vi "CPP_SolAE_Plot_Many_Channels.vi"() -> (5 "Plug in titles":string[](array[string]), 7 "Plug in values":string[](array[string]))   [LabVIEW 2021]
uses:
  <vilib>/Analysis/2dsp.llb/Decimate (single shot, DBL).vi
  07834b75-344c-4d4c-a66e-07bf327eec95.vi
  Globals/Meas_global.vi
  <vilib>/Analysis/NI_AALBase.lvlib
  <vilib>/Analysis/NI_AALPro.lvlib
panel:
  in  "decimating factor":i32=400
  in  "Tab Control":T1(tab)
  out "XY Graph":cluster{"Time (s)":dbl[], "Voltage":dbl[]}[](graph)
  out "XY Graph 2":cluster{"Time (s)":dbl[], "Voltage":dbl[]}[](graph)
  out "XY Graph 3":cluster{"Time (s)":dbl[], "Voltage":dbl[]}[](graph)
  out "XY Graph 4":cluster{"Time (s)":dbl[], "Voltage":dbl[]}[](graph)
  out "XY Graph 5":cluster{"Time (s)":dbl[], "Voltage":dbl[]}[](graph)
  out "XY Graph 6":cluster{"Time (s)":dbl[], "Voltage":dbl[]}[](graph)
  in  "Display:":enum16{"Show All", "My Choice", "Hide All"}(ring)
  in  "Plot:":enum16{"Eng. Units", "Voltages"}(ring)
  # "Channel"
  # "Value"
  # "Voltage"
  # "StdDev(V)"
  # "Name"
  # "Symbol"
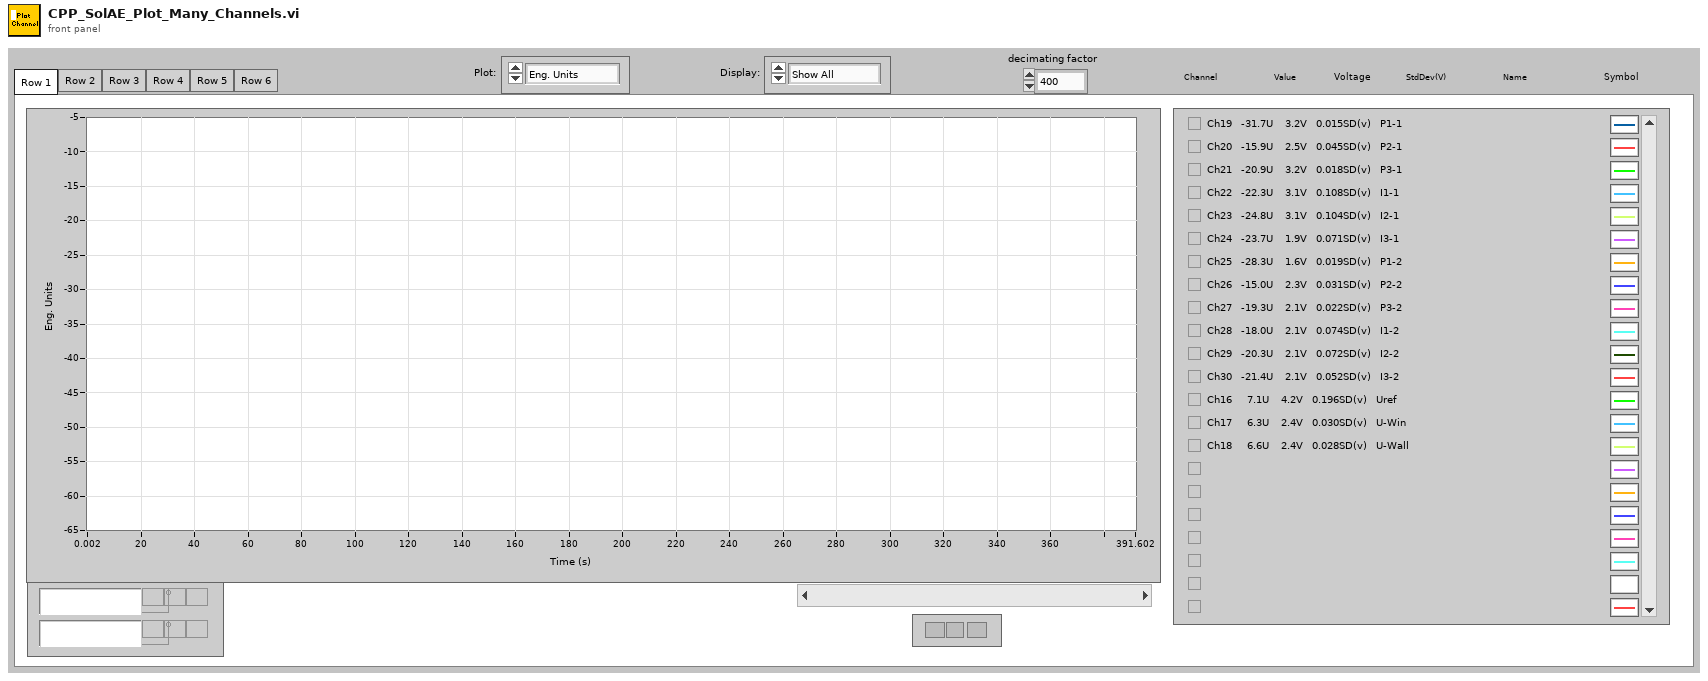
[diagram p1: front panel]
types:
  T1 = enum32{"Row 1", "Row 2", "Row 3", "Row 4", "Row 5", "Row 6"}
  T2 = typedef "Analysis_info_cluster.ctl" = cluster{"Colour":u32, "Inst type":T3, "Inst name":string, "Symbol":string, "Code name":string, "Extra Info":string, "Inst Array":T4, "Extra Titles":string[], "Extra Values":string[], "U":dbl, "u^2":dbl, "u^3":dbl, "u^4":dbl, "Skew_u":dbl, "Kurt_u":dbl, "Sd Error in Mean":dbl, "% u'/U":dbl, "X":dbl, "Y":dbl, "Z":dbl, "Timescale integral Estimate":dbl, "Sd Error in Variance":dbl, "Calib File":path, "Calib Constants":dbl[], "Output Position":bool, "Stats":enum16{"None", "Basic", "Full"}, "Av Sampling Rate":dbl, "Av No of Samples":dbl, "Total Meas Time (s)":dbl, "ADAM Ch Name":string, "Max value":dbl, "Min value":dbl, "Req Sample Rate Hz":dbl, "Sync Delay Time (s)":dbl, "Ch No":i16, "Device":string, "Use Latest Calib":bool, "Port":string, "Metadata Ch Names":string[], "Metadata Ch Values":string[], "Label":string}
  T3 = typedef "Inst_type.ctl" = enum16{"Raw voltage", "Raw with zero offsetting", "Propeller anemometer", "Pressure Transducer", "Pitot-static tube", "Hot wire", "Cross wire 1", "Cross wire 2", "Generic Linear", "Generic Polynomial", "Generic BackPoly", "Fast FID", "Thermocouple", "Cold wire", "Pulsed Wire", "LDA Vel", "LDA Tran time", "LDA Arr time", "Microphone"}
  T4 = typedef "Instrument_Array.ctl" = enum16{"PWA", "LDA", "Analogue"}
  T5 = typedef "Time_Trace_Cluster.ctl" = cluster{"Weighting":dbl[], "Voltage":dbl[], "Eng Values":dbl[]}
  T6 = cluster{"Decimated Array":dbl[], "Decimated Array":dbl[]}
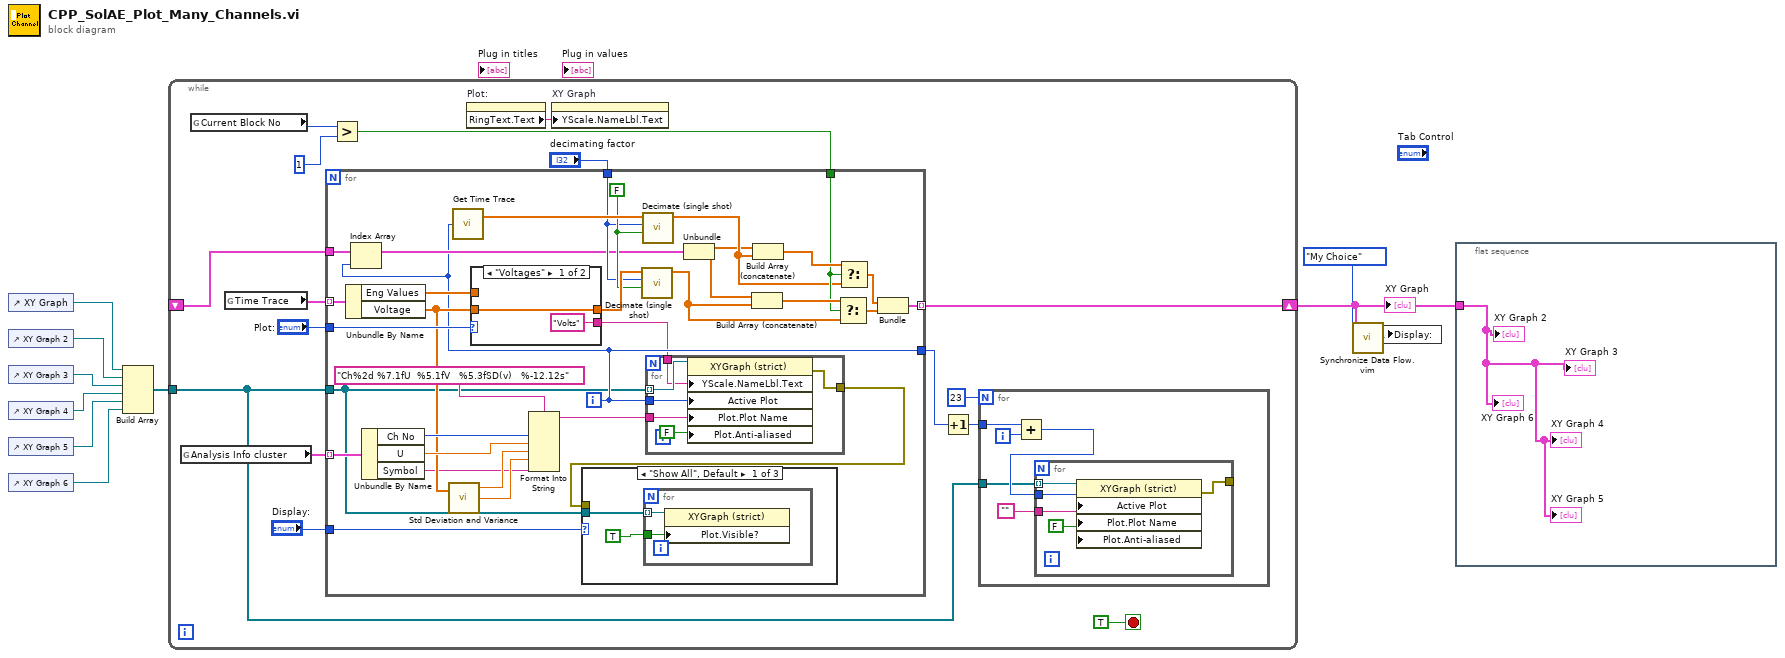
[diagram p0: block diagram]
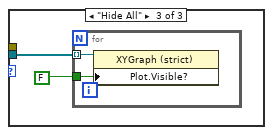
[diagram p3: hidden frame]
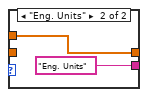
[diagram p4: hidden frame]
diagram:
  n1 = control-ref of="XY Graph"() -> (w7:refnum<vi>)
  n2 = control-ref of="XY Graph 2"() -> (w6:refnum<vi>)
  n3 = control-ref of="XY Graph 3"() -> (w5:refnum<vi>)
  n4 = control-ref of="XY Graph 4"() -> (w4:refnum<vi>)
  n5 = control-ref of="XY Graph 5"() -> (w3:refnum<vi>)
  n6 = control-ref of="XY Graph 6"() -> (w2:refnum<vi>)
  n7 = Build Array(w7, w6, w5, w4, w3, w2) -> (w1:refnum<vi>[])
  n8 = while {
    shift-right: [w21] -> w8
    shift-left: _ -> [w13]
    tunnel: w1 -> [w11]
    stop <- TRUE stop-if-true
    n9 = global read "Meas_global.vi" "Analysis Info cluster"() -> (w26:T2[])
    n10 = global read "Meas_global.vi" "Current Block No"() -> (w16:i32)
    n11 = global read "Meas_global.vi" "Time Trace"() -> (w23:T5[])
    n12 = Greater?(x=w16, y=1) -> (0:w12:bool)
    n13 = for {
      tunnel: [w51] -> w21 mode=indexing
      tunnel: w26 -> [w69] mode=indexing
      tunnel: "Plot:" -> [w68]
      tunnel: "Display:" -> [w57]
      tunnel: w23 -> [w56] mode=indexing
      tunnel: [w39] -> w19
      tunnel: "decimating factor" -> [w52]
      tunnel: w13 -> [w50]
      tunnel: w12 -> [w45]
      tunnel: w11 -> [w38]
      i -> [w39]
      w53 = FALSE ("averaging")
      n14 = Unbundle By Name(w56) -> ("Eng Values"=w63:dbl[], "Voltage"=w62:dbl[])
      n15 = Index Array(array=w50, index=w39) -> (element=w40:T6)
      n16 = Unbundle By Name(w69) -> ("Ch No"=w67:i16, "U"=w66:dbl, "Symbol"=w59:string)
      n17 = call <vilib>:"Std Deviation and Variance.vi"("X"=w62) -> ("mean"=w61:dbl, "standard deviation"=w60:dbl)  [unwired: 1 in, 1 out]
      n18 = call "Get Time Trace.vi"("Channel Index"=w39) -> ("Time (s)"=w55:dbl[])  [unwired: 1 out]
      n19 = case shown="\"Voltages\"" w68 {
        tunnel: [w85 w87] -> w54
        tunnel: w62 -> [w85 _]
        tunnel: w63 -> [_ w87]
        tunnel: ["Volts" "Eng. Units"] -> w37
        frame "Voltages" {
        }
        frame "Eng. Units" {
        }
      }
      n20 = Format Into String(format string="Ch%2d %7.1fU  %5.1fV   %5.3fSD(v)   %-12.12s", w67, w66, w61, w60, w59) -> (resulting string=w65:string)  [unwired: 2 in, 1 out]
      n21 = call-poly <vilib>:"Decimate (single shot).vi"("averaging"=w53, "decimating factor"=w52, "X"=w54) -> ("Decimated Array"=w47:dbl[])  [unwired: 7 in, 1 out]
      n22 = call-poly <vilib>:"Decimate (single shot).vi"("averaging"=w53, "decimating factor"=w52, "X"=w55) -> ("Decimated Array"=w42:dbl[])  [unwired: 7 in, 1 out]
      n23 = for {
        tunnel: w65 -> [w75]
        tunnel: [w74] -> w58
        tunnel: w39 -> [w71]
        tunnel: w38 -> [w73] mode=indexing
        tunnel: w37 -> [w70]
        n24 = property class="XYGraph (strict)"(reference=w73, "YScale.NameLbl.Text"=w70, "Active Plot"=w71, "Plot.Plot Name"=w75, "Plot.Anti-aliased"=FALSE) -> (error out=w74:errorcluster)  [unwired: 1 in, 1 out]
      }
      n25 = case shown="\"Show All\", Default" w57 {
        tunnel: w58 -> [_ _ _]
        tunnel: w38 -> [w76 _ w80]
        frame "Show All", Default {
          n26 = for {
            tunnel: TRUE ("Plot.Visible") -> [w79]
            tunnel: w76 -> [w78] mode=indexing
            n27 = property class="XYGraph (strict)"(reference=w78, "Plot.Visible?"=w79) -> ()  [unwired: 1 in, 2 out]
          }
        }
        frame "My Choice" {
        }
        frame "Hide All" {
          n28 = for {
            tunnel: FALSE ("Plot.Visible") -> [w83]
            tunnel: w80 -> [w82] mode=indexing
            n29 = property class="XYGraph (strict)"(reference=w82, "Plot.Visible?"=w83) -> ()  [unwired: 1 in, 2 out]
          }
        }
      }
      n30 = Unbundle(w40) -> ("Decimated Array"=w41:dbl[], "Decimated Array"=w49:dbl[])
      n31 = Build Array (concatenate)(w49, w47) -> (w46:dbl[])
      n32 = Build Array (concatenate)(w41, w42) -> (w48:dbl[])
      n33 = Select(t=w46, s=w45, f=w47) -> (s? t:f=w44:dbl[])
      n34 = Select(t=w48, s=w45, f=w42) -> (s? t:f=w43:dbl[])
      n35 = Bundle("Decimated Array"=w43, "Decimated Array"=w44) -> (w51:T6)  [unwired: 1 in]
    }
    n36 = property on="Plot:" class="Enum (strict)"() -> ("RingText.Text"=w22:string)  [unwired: 2 in, 2 out]
    n37 = property on="XY Graph" class="XYGraph (strict)"("YScale.NameLbl.Text"=w22) -> ()  [unwired: 2 in, 2 out]
    n38 = Increment(x=w19) -> (x+1=w20:i32)
    n39 = for {
      N: 23 -> [_]
      tunnel: w20 -> [w30]
      tunnel: w11 -> [w27]
      i -> [w31]
      n40 = Add(x=w30, y=w31) -> (x+y=w28:i32)
      n41 = for {
        tunnel: "" -> [w35]
        tunnel: [w34] -> _
        tunnel: w28 -> [w36]
        tunnel: w27 -> [w33] mode=indexing
        n42 = property class="XYGraph (strict)"(reference=w33, "Active Plot"=w36, "Plot.Plot Name"=w35, "Plot.Anti-aliased"=FALSE) -> (error out=w34:errorcluster)  [unwired: 1 in, 1 out]
      }
    }
  }
  "XY Graph" <- w8
  n43 = call "Synchronize Data Flow.vim"("input 2"=enum16{"Show All", "My Choice", "Hide All"}."My Choice" ("show"), "input 1"=w8) -> ("output 2"=w9:enum16{"Show All", "My Choice", "Hide All"})  [unwired: 2 in, 3 out]
  n44 = local write "Display:"(w9) -> ()
  n45 = flat-sequence {
    tunnel: w8 -> [w88]
    frame #0 {
      "XY Graph 2" <- w88
      "XY Graph 4" <- w88
      "XY Graph 5" <- w88
      "XY Graph 6" <- w88
      "XY Graph 3" <- w88
    }
  }
